vi "LS 336 T Ramp Text Out.vi"(1 "Timed Ramp":T1={"VISA Resource Name"="", "extra wait"=1, "start"=1.0, "end"=4.0, "Sweep Time (H:M:S)"=10.0, "Log Linear"=FALSE, "Heater Range"=enum."OFF", "Loop"=FALSE} {"Sweep Time (H:M:S)" format="%<%H:%M:%S>t"; "extra wait" min=0; "start" format="%#.7e"; "end" format="%#.7e"}) -> (0 "Command text":string[][](array[string]))   [LabVIEW 2019]
uses:
  LS 336 T Ramp.ctl
panel:
  out "Heater Range 2":string
  out "Heater Range":enum16{"OFF", "LOW", "MEIDUM", "HIGH"}(ring)
  out "Sweep Time (H:M:S)":dbl
  out "String Cluster":T2
  # "LS 336 Temp Setpoint (K) Ramp"
  # "Log"
  # "End Temp (K)"
  # "Sweep Time (HH:MM:SS)"
  # "Start Temp (K)"
  # "Linear"
  # "seconds"
  # "AND wait extra"
  # "Which Heater to control?"
  # "VISA Name"
  # "Loop 2\n(Probe / 3He Pot)"
  # "Heater Range"
  # "Loop 1\n(Sorb / VTI)"
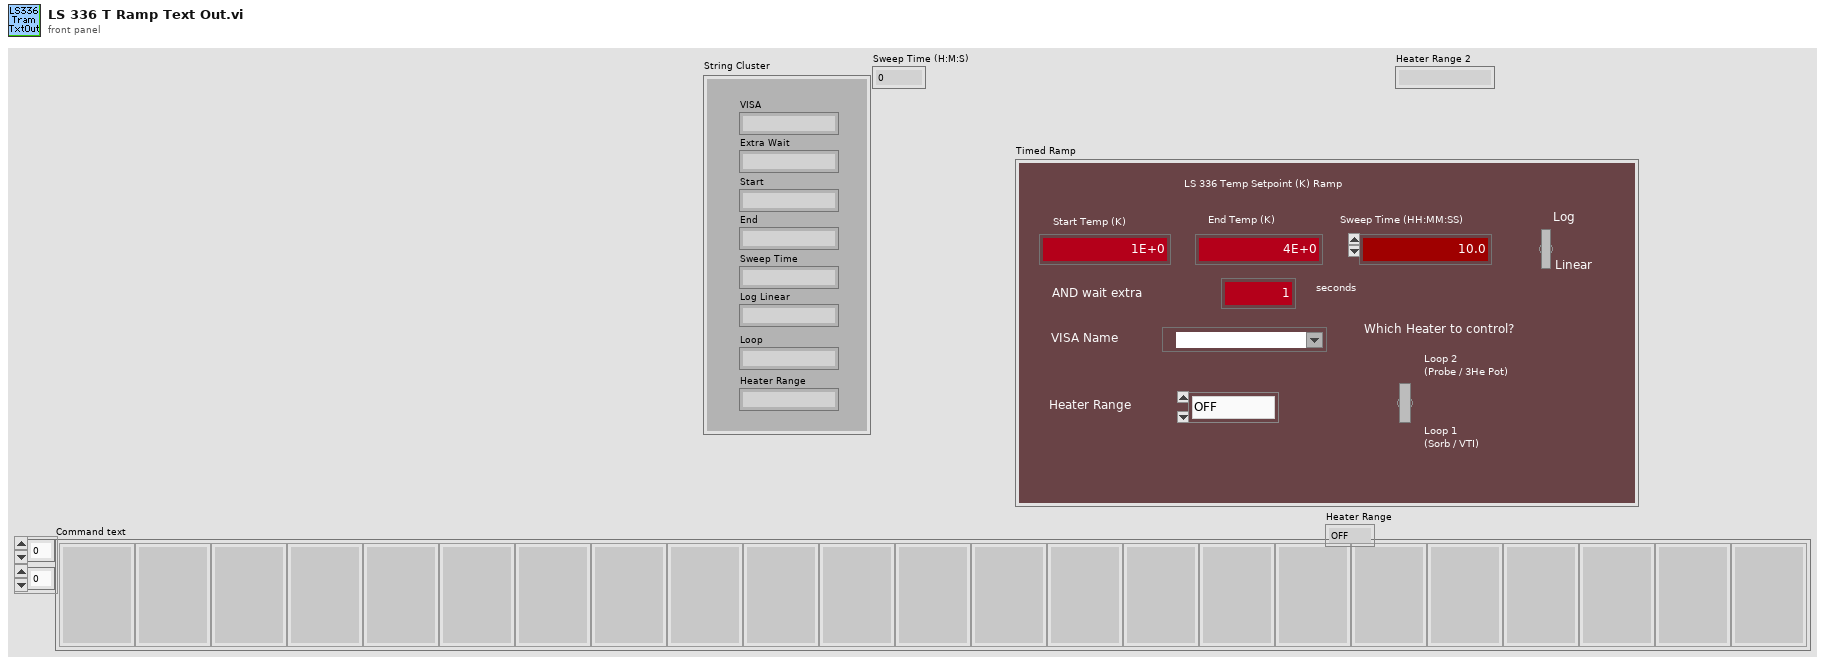
[diagram p1: front panel]
types:
  T1 = typedef "LS 336 T Ramp.ctl" = cluster{"VISA Resource Name":refnum<visa-resource-name>, "extra wait":i32, "start":dbl, "end":dbl, "Sweep Time (H:M:S)":dbl, "Log Linear":bool, "Heater Range":enum16{"OFF", "LOW", "MEIDUM", "HIGH"}, "Loop":bool}
  T2 = cluster{"VISA":string, "Extra Wait":string, "Start":string, "End":string, "Sweep Time":string, "Log Linear":string, "Loop":string, "Heater Range":string}
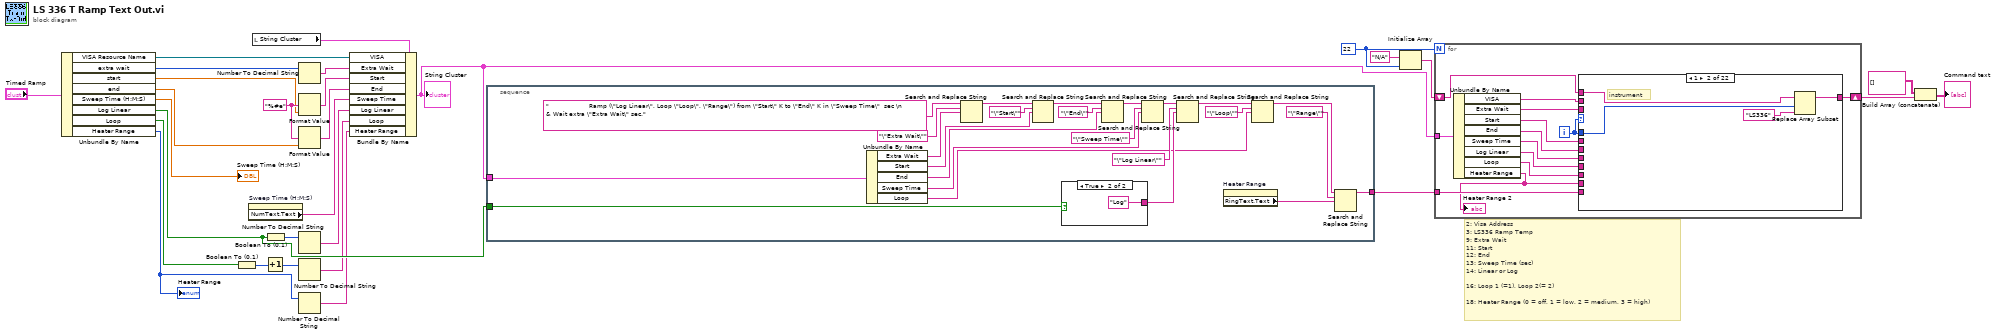
[diagram p0: block diagram]
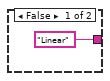
[diagram p2: hidden frame]
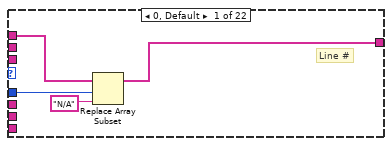
[diagram p3: hidden frame]
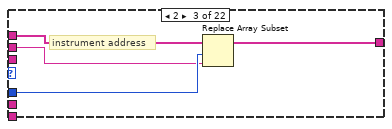
[diagram p4: hidden frame]
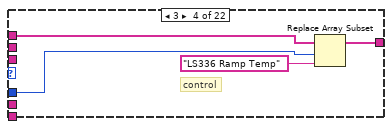
[diagram p5: hidden frame]
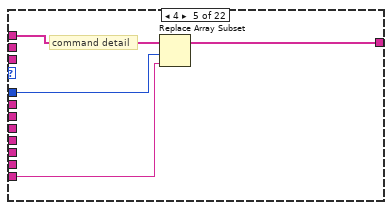
[diagram p6: hidden frame]
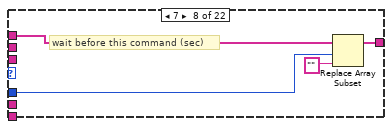
[diagram p9: hidden frame]
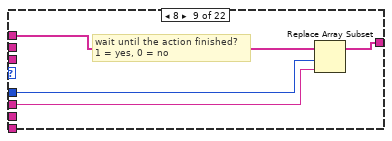
[diagram p10: hidden frame]
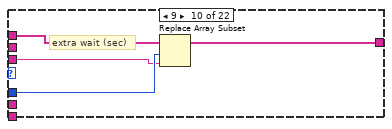
[diagram p11: hidden frame]
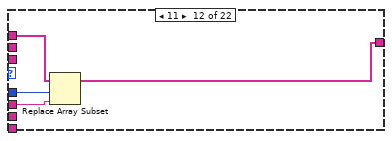
[diagram p13: hidden frame]
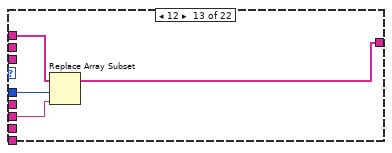
[diagram p14: hidden frame]
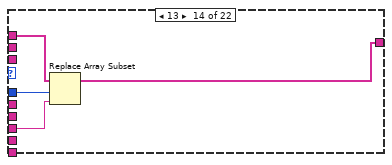
[diagram p15: hidden frame]
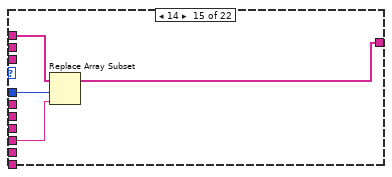
[diagram p16: hidden frame]
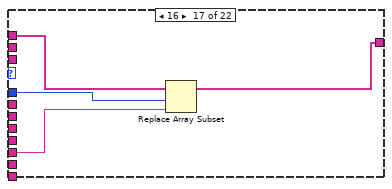
[diagram p18: hidden frame]
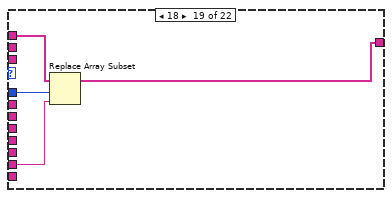
[diagram p20: hidden frame]
diagram:
  w18 = "%#e" ("format string")
  w26 = 22
  # "2: Visa Address\n3: LS336 Ramp Temp\n9: Extra Wait\n11: Start\n12: End\n13: Sweep Time (sec)\n14: Linear or Log\n\n16: Loop 1 (=1), Loop 2(= 2)\n\n18: Heater Range (0 = off, 1 = low, 2 = medium, 3 = high)"
  n1 = Unbundle By Name("Timed Ramp") -> ("VISA Resource Name"=w11:refnum<visa-resource-name>, "extra wait"=w13:i32, "start"=w16:dbl, "end"=w17:dbl, "Sweep Time (H:M:S)"=→"Sweep Time (H:M:S)":dbl, "Log Linear"=w9:bool, "Loop"=w7:bool, "Heater Range"=w5:enum16{"OFF", "LOW", "MEIDUM", "HIGH"})
  "Heater Range" <- w5
  n2 = Boolean To (0,1)(Boolean=w7) -> (0, 1=w2:i16)
  n3 = property on="Sweep Time (H:M:S)" class="DigNum (strict)"() -> ("NumText.Text"=w19:string)  [unwired: 2 in, 2 out]
  n4 = local read "String Cluster"() -> (w23:T2)
  n5 = Boolean To (0,1)(Boolean=w9) -> (0, 1=w10:i16)
  n6 = Increment(x=w2) -> (x+1=w3:i16)
  n7 = Number To Decimal String(number=w13) -> (decimal integer string=w12:string)  [unwired: 1 in]
  n8 = Format Value(format string=w18, value (0)=w16) -> (output string=w15:string)  [unwired: 1 in]
  n9 = Format Value(format string=w18, value (0)=w17) -> (output string=w14:string)  [unwired: 1 in]
  n10 = Number To Decimal String(number=w10) -> (decimal integer string=w8:string)  [unwired: 1 in]
  n11 = Number To Decimal String(number=w3) -> (decimal integer string=w6:string)  [unwired: 1 in]
  n12 = Number To Decimal String(number=w5) -> (decimal integer string=w4:string)  [unwired: 1 in]
  n13 = Bundle By Name(cluster=w23, "VISA"=w11, "Extra Wait"=w12, "Start"=w15, "End"=w14, "Sweep Time"=w19, "Log Linear"=w8, "Loop"=w6, "Heater Range"=w4) -> (w21:T2)
  "String Cluster" <- w21
  n14 = stacked-sequence {
    tunnel: [w30] -> w22
    tunnel: w21 -> [w45]
    tunnel: w9 -> [w37]
    frame #0 {
      n15 = Unbundle By Name(w45) -> ("Extra Wait"=w44:string, "Start"=w43:string, "End"=w42:string, "Sweep Time"=w41:string, "Loop"=w35:string)
      n16 = Search and Replace String(input string="                    Ramp (\"Log Linear\", Loop \"Loop\", \"Range\") from \"Start\" K to \"End\" K in \"Sweep Time\"  sec \n                    & Wait extra \"Extra Wait\" sec.", search string="\"Extra Wait\"", replace string=w44) -> (result string=w51:string)  [unwired: 5 in, 3 out]
      n17 = Search and Replace String(input string=w51, search string="\"Start\"", replace string=w43) -> (result string=w52:string)  [unwired: 5 in, 3 out]
      n18 = case shown="True" w37 {
        tunnel: ["Linear" "Log"] -> w40
        frame False {
        }
        frame True {
        }
      }
      n19 = Search and Replace String(input string=w52, search string="\"End\"", replace string=w42) -> (result string=w53:string)  [unwired: 5 in, 3 out]
      n20 = Search and Replace String(input string=w53, search string="\"Sweep Time\"", replace string=w41) -> (result string=w39:string)  [unwired: 5 in, 3 out]
      n21 = Search and Replace String(input string=w39, search string="\"Log Linear\"", replace string=w40) -> (result string=w36:string)  [unwired: 5 in, 3 out]
      n22 = property on="Heater Range" class="Enum (strict)"() -> ("RingText.Text"=w31:string)  [unwired: 2 in, 2 out]
      n23 = Search and Replace String(input string=w36, search string="\"Loop\"", replace string=w35) -> (result string=w33:string)  [unwired: 5 in, 3 out]
      n24 = Search and Replace String(input string=w33, search string="\"Range\"", replace string=w31) -> (result string=w30:string)  [unwired: 5 in, 3 out]
    }
  }
  n25 = Initialize Array("N/A", w26) -> (w25:string[])
  n26 = for {
    N: w26 -> [_]
    shift-right: [w66] -> w24
    shift-left: w25 -> [w67]
    tunnel: w22 -> [w65]
    tunnel: w21 -> [w64]
    i -> [w68]
    n27 = Unbundle By Name(w64) -> ("VISA"=w61:string, "Extra Wait"=w60:string, "Start"=w63:string, "End"=w62:string, "Sweep Time"=w59:string, "Log Linear"=w58:string, "Loop"=w57:string, "Heater Range"=w56:string)
    "Heater Range 2" <- w56
    n28 = case shown="1" w68 {
      tunnel: w68 -> [w71 w75 w80 w82 w87 _ _ w92 w96 w100 _ w105 w109 w115 w117 _ w122 _ w127 _ _ _]
      tunnel: w67 -> [w72 w74 w79 w83 w88 w89 w90 w94 w98 w102 w103 w106 w111 w113 w119 w120 w124 w125 w129 w130 w131 w132]
      tunnel: [w69 w73 w78 w81 w86 w89 w90 w93 w97 w101 w103 w107 w110 w112 w118 w120 w123 w125 w128 w130 w131 w132] -> w66
      tunnel: w65 -> [_ _ _ _ w85 _ _ _ _ _ _ _ _ _ _ _ _ _ _ _ _ _]
      tunnel: w63 -> [_ _ _ _ _ _ _ _ w95 _ _ w104 _ _ _ _ _ _ _ _ _ _]
      tunnel: w62 -> [_ _ _ _ _ _ _ _ _ _ _ _ w108 _ _ _ _ _ _ _ _ _]
      tunnel: w61 -> [_ _ w77 _ _ _ _ _ _ _ _ _ _ _ _ _ _ _ _ _ _ _]
      tunnel: w60 -> [_ _ _ _ _ _ _ _ _ w99 _ _ _ _ _ _ _ _ _ _ _ _]
      tunnel: w59 -> [_ _ _ _ _ _ _ _ _ _ _ _ _ w114 _ _ _ _ _ _ _ _]
      tunnel: w58 -> [_ _ _ _ _ _ _ _ _ _ _ _ _ _ w116 _ _ _ _ _ _ _]
      tunnel: w57 -> [_ _ _ _ _ _ _ _ _ _ _ _ _ _ _ _ w121 _ _ _ _ _]
      tunnel: w56 -> [_ _ _ _ _ _ _ _ _ _ _ _ _ _ _ _ _ _ w126 _ _ _]
      frame 0, Default {
        # "Line #"
        n29 = Replace Array Subset(array=w72, new element="N/A", index=w71) -> (w69:string[])
      }
      frame 1 {
        # "instrument"
        n30 = Replace Array Subset(array=w74, new element="LS336", index=w75) -> (w73:string[])
      }
      frame 2 {
        # "instrument address"
        n31 = Replace Array Subset(array=w79, new element=w77, index=w80) -> (w78:string[])
      }
      frame 3 {
        # "control"
        n32 = Replace Array Subset(array=w83, new element="LS336 Ramp Temp", index=w82) -> (w81:string[])
      }
      frame 4 {
        # "command detail"
        n33 = Replace Array Subset(array=w88, new element=w85, index=w87) -> (w86:string[])
      }
      frame 5 {
        # "in  case 1"
      }
      frame 6 {
        # "in case 2"
      }
      frame 7 {
        # "wait before this command (sec)"
        n34 = Replace Array Subset(array=w94, new element="" ("new element/subarray"), index=w92) -> (w93:string[])
      }
      frame 8 {
        # "wait until the action finished?\n1 = yes, 0 = no"
        n35 = Replace Array Subset(array=w98, new element=w95, index=w96) -> (w97:string[])
      }
      frame 9 {
        # "extra wait (sec)"
        n36 = Replace Array Subset(array=w102, new element=w99, index=w100) -> (w101:string[])
      }
      frame 10 {
      }
      frame 11 {
        n37 = Replace Array Subset(array=w106, new element=w104, index=w105) -> (w107:string[])
      }
      frame 12 {
        n38 = Replace Array Subset(array=w111, new element=w108, index=w109) -> (w110:string[])
      }
      frame 13 {
        n39 = Replace Array Subset(array=w113, new element=w114, index=w115) -> (w112:string[])
      }
      frame 14 {
        n40 = Replace Array Subset(array=w119, new element=w116, index=w117) -> (w118:string[])
      }
      frame 15 {
      }
      frame 16 {
        n41 = Replace Array Subset(array=w124, new element=w121, index=w122) -> (w123:string[])
      }
      frame 17 {
      }
      frame 18 {
        n42 = Replace Array Subset(array=w129, new element=w126, index=w127) -> (w128:string[])
      }
      frame 19 {
      }
      frame 20 {
      }
      frame 21 {
      }
    }
  }
  n43 = Build Array (concatenate)(string[][] [], w24) -> (→"Command text":string[][])
